vi "Build CHM.vi"   [LabVIEW 2020]
uses:
  <vilib>/Utility/config.llb/Read Key (String).vi
  <vilib>/Utility/config.llb/Read Key (Path).vi
  vi.lib/NI/Compiled HTML Menu Tool/CHM Generator/CHM Generator.lvclass
  <vilib>/Utility/config.llb/NI_LVConfig.lvlib
types:
  T1 = typedef "NI_LVConfig.lvlib/Config Data RefNum.ctl" = refnum<k1>
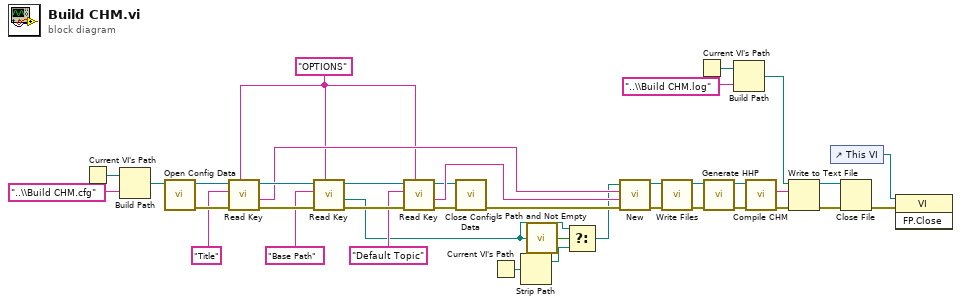
[diagram p0: block diagram]
diagram:
  w19 = "OPTIONS" ("section")
  n1 = Current VI's Path() -> (path=w18:path)
  n2 = Build Path(base path=w18, name or relative path="..\\Build CHM.cfg") -> (appended path=w16:path)
  n3 = call <vilib>:"Open Config Data.vi"("configuration file path"=w16) -> ("error out"=w31:errorcluster, "refnum"=w32:T1)  [unwired: 8 in, 1 out]
  n4 = call-poly <vilib>:"Read Key.vi"("section"=w19, "error in (no error)"=w31, "key"="Title", "refnum"=w32) -> ("error out"=w29:errorcluster, "value"=w26:string, "refnum out"=w28:T1)  [unwired: 4 in, 1 out]
  n5 = call-poly <vilib>:"Read Key.vi"("section"=w19, "error in (no error)"=w29, "key"="Base Path", "refnum"=w28) -> ("error out"=w25:errorcluster, "value"=w2:path, "refnum out"=w24:T1)  [unwired: 4 in, 1 out]
  n6 = call-poly <vilib>:"Read Key.vi"("section"=w19, "error in (no error)"=w25, "key"="Default Topic", "refnum"=w24) -> ("error out"=w21:errorcluster, "value"=w22:string, "refnum out"=w20:T1)  [unwired: 4 in, 1 out]
  n7 = call <vilib>:"Close Config Data.vi"("error in (no error)"=w21, "refnum"=w20) -> ("error out"=w6:errorcluster)  [unwired: 8 in, 1 out]
  n8 = Current VI's Path() -> (path=w4:path)
  n9 = Strip Path(path=w4) -> (stripped path=w3:path)  [unwired: 1 out]
  n10 = call <vilib>:"Is Path and Not Empty.vi"("path"=w2) -> ("Is Path and Not Empty?"=w5:bool)  [unwired: 4 in]
  n11 = Select(t=w2, s=w5, f=w3) -> (s? t:f=w1:path)
  n12 = call "New.vi"("error in (no error)"=w6, "Default topic"=w22, "Title"=w26, "Base Path"=w1) -> ("error out"=w37:errorcluster, "CHM Generator out"=w38:refnum<class "CHM Generator.lvclass">)  [unwired: 6 in]
  n13 = call-dynamic "Write Files.vi"("error in (no error)"=w37, "CHM Generator in"=w38) -> ("error out"=w36:errorcluster, "CHM Generator out"=w35:refnum<class "CHM Generator.lvclass">)  [unwired: 8 in]
  n14 = Current VI's Path() -> (path=w15:path)
  n15 = call-dynamic "Generate HHP.vi"("error in (no error)"=w36, "CHM Generator in"=w35) -> ("error out"=w33:errorcluster, "CHM Generator out"=w34:refnum<class "CHM Generator.lvclass">)  [unwired: 8 in]
  n16 = Build Path(base path=w15, name or relative path="..\\Build CHM.log") -> (appended path=w13:path)
  n17 = call "Compile CHM.vi"("error in (no error)"=w33, "CHM Generator in"=w34) -> ("error out"=w9:errorcluster, "standard output"=w12:string)  [unwired: 7 in, 1 out]
  n18 = Write to Text File(file (use dialog)=w13, text=w12, error in=w9) -> (refnum out=w10:refnum<file>, error out=w11:errorcluster)  [unwired: 1 in, 1 out]
  n19 = control-ref of="This VI"() -> (w8:refnum<vi>)
  n20 = Close File(refnum=w10, error in=w11) -> (error out=w7:errorcluster)  [unwired: 1 out]
  n21 = invoke class="VI" method="FP.Close"(reference=w8, error in=w7) -> ()  [unwired: 1 in, 3 out]
